vi "solar_read QTimerNames.vi"(8 "error in (no error)":errorcluster, 11 "solar in":refnum<class "solar.lvclass">) -> (0 "error out":errorcluster, 2 "QTimers":string[](array[string]), 3 "solar out":refnum<class "solar.lvclass">)   [LabVIEW 2018, in "solar.lvclass"]
doc: "This returns all QTimers registered with this interface."
uses:
  solar.lvclass
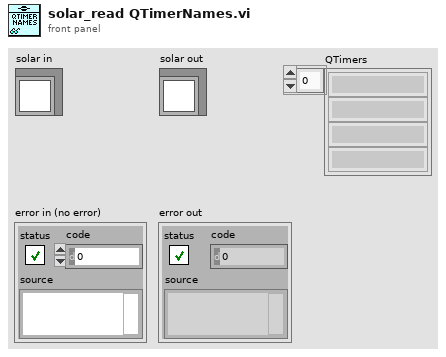
[diagram p1: front panel]
types:
  T1 = typedef "solar_ctl SOLAR Refnum.ctl" = refnum<k1>
  T2 = typedef "solar_ctl SOLAR Global.ctl" = cluster{"Targets":T3[], "AppDir":path, "solar.ini":path, "ConfigsDir":path, "CosmosDir":path, "LogsDir":path, "ExePath":path, "ExeVersion":string, "PartNum":string, "AppSetup":string, "Title":string, "Main.ini":path, "Temp.ini":path, "vSOLAR":string, "Splash.png":string, "SplashWait":i32, "SOLARUE":refnum<user-event>, "VoyagerRefnum":T4, "QTimerRefnum":T5}
  T3 = typedef "solar_ctl Target Global.ctl" = cluster{"Target":string, "Q":refnum<queue>, "UE":refnum<user-event>, "VI":refnum<vi>, "Menu":refnum<k9>, "Data":refnum<data-value>, "Attributes":variant}
  T4 = typedef "solar_voy_ctl Voyager Refnum.ctl" = refnum<k1>
  T5 = typedef "solar_qtimer_ctl Refnum.ctl" = refnum<k1>
  T6 = typedef "solar_qtimer_ctl QTimer.ctl" = cluster{"Settings":T7, "Queue":refnum<queue>, "QTimerQ":refnum<queue>, "VI Refnum":refnum<vi>}
  T7 = typedef "solar_qtimer_ctl QTimer Settings.ctl" = cluster{"QTimer":string, "Delay":i32, "Start":bool, "EnQ_Type":enum8{"Normal", "Priority", "IgnoreIfExists"}, "Messages":cluster{"MSG":string, "DATA":variant}[]}
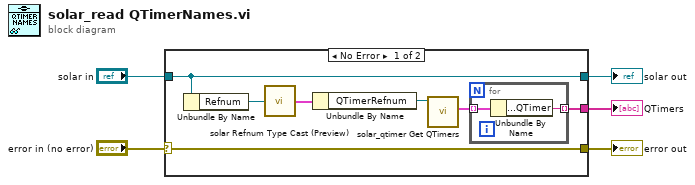
[diagram p0: block diagram]
diagram:
  n1 = case shown="No Error" "error in (no error)" {
    selector: "error in (no error)" -> [w10 w16]
    tunnel: "solar in" -> [w9 w15]
    tunnel: [w10 w16] -> w4
    tunnel: [w9 w15] -> w2
    tunnel: [w6 _] -> w1
    frame No Error {
      n2 = Unbundle By Name(w9) -> ("Refnum"=w12:T1)
      n3 = call "solar Refnum Type Cast (Preview).vi"("Refnum"=w12) -> ("SOLAR"=w11:T2)  [unwired: 8 in]
      n4 = Unbundle By Name(w11) -> ("QTimerRefnum"=w8:T5)
      n5 = call "solar_qtimer Get QTimers.vi"("QTimer Refnum"=w8) -> ("QTimers"=w7:T6[])  [unwired: 8 in, 2 out]
      n6 = for {
        tunnel: w7 -> [w14] mode=indexing
        tunnel: [w13] -> w6 mode=indexing
        n7 = Unbundle By Name(w14) -> ("Settings.QTimer"=w13:string)
      }
    }
    frame Error {
    }
  }
  "error out" <- w4
  "solar out" <- w2
  "QTimers" <- w1
